vi "temp_directory_delete.vi"(8 "error in (no error)":errorcluster) -> (0 "error out":errorcluster)   [LabVIEW 2015, in "lv-post-installer.lvlib"]
uses:
  lv-post-installer.lvlib
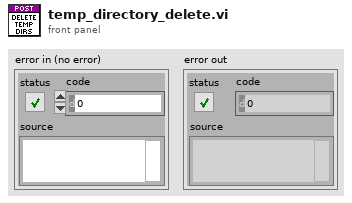
[diagram p1: front panel]
types:
  T1 = typedef "lv-post-installer.lvlib/temp_dir_config.ctl" = cluster{"root_folder":path, "prefix":string}
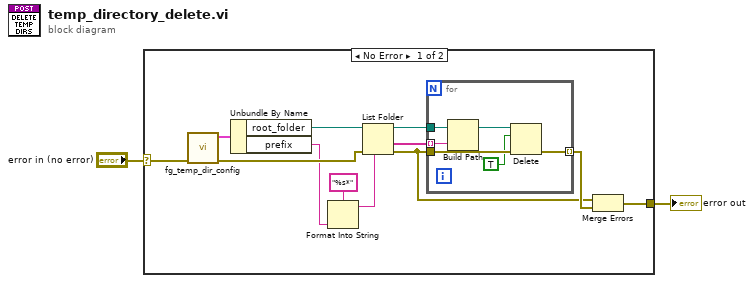
[diagram p0: block diagram]
diagram:
  n1 = case shown="No Error" "error in (no error)" {
    selector: "error in (no error)" -> [w13 w21]
    tunnel: [w7 w21] -> w1
    frame No Error {
      n2 = call "fg_temp_dir_config.vi"("error in (no error)"=w13) -> ("error out"=w14:errorcluster, "temp_dir_config"=w12:T1)  [unwired: 9 in]
      n3 = Unbundle By Name(w12) -> ("root_folder"=w11:path, "prefix"=w6:string)
      n4 = Format Into String(format string="%s*", w6) -> (resulting string=w5:string)  [unwired: 2 in, 1 out]
      n5 = List Folder(path=w11, pattern=w5, error in=w14) -> (path out=w10:path, folder names=w9:string[], error out=w3:errorcluster)  [unwired: 1 in, 1 out]
      n6 = for {
        tunnel: w3 -> [w18]
        tunnel: w10 -> [w20]
        tunnel: w9 -> [w19] mode=indexing
        tunnel: [w17] -> w8 mode=indexing
        n7 = Build Path(base path=w20, name or relative path=w19) -> (appended path=w15:path)
        n8 = Delete(path (use dialog)=w15, entire hierarchy (F)=TRUE, error in=w18) -> (error out=w17:errorcluster)  [unwired: 2 in, 2 out]
      }
      n9 = Merge Errors(w3, w8) -> (w7:errorcluster)
    }
    frame Error {
    }
  }
  "error out" <- w1
